vi "Do.vi"(8 "error in (no error)":errorcluster, 10 "Actor in":refnum<class "Actor.lvclass">, 11 "Stage Printing Loop Msg in":refnum<class "Stage Printing Loop Msg.lvclass">) -> (0 "error out":errorcluster, 2 "Actor out":refnum<class "Actor.lvclass">)   [LabVIEW 2018, in "Stage Printing Loop Msg.lvclass"]
doc: "This VI delivers the message to the actor by calling the appropriate method(s) on the actor."
uses:
  Stage Printing Loop Msg.lvclass
  <vilib>/ActorFramework/Actor/Actor.lvclass
  Stage/Stage.lvclass
  C:/Program Files/National Instruments/LabVIEW 2018/vi.lib/ActorFramework/Actor/Actor.lvclass
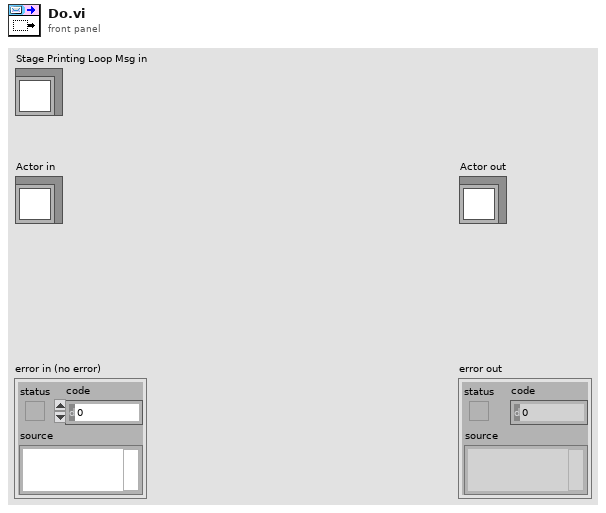
[diagram p1: front panel]
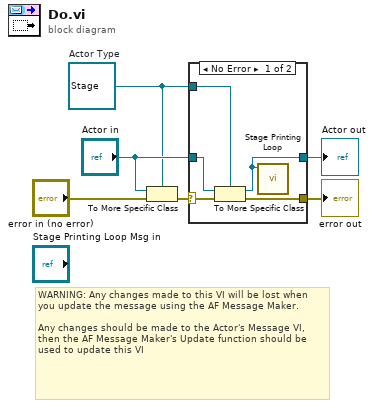
[diagram p0: block diagram]
diagram:
  w1 = refnum<class "Stage.lvclass"> refnum  # Actor Type
  # "WARNING: Any changes made to this VI will be lost when you update the message using the AF Message Maker.\n\nAny changes should be made to the Actor's Message VI, then the AF Message Maker's Update function should be used to update this VI"
  n1 = To More Specific Class(target class=w1, reference="Actor in", error in="error in (no error)") -> (error out=w5:errorcluster)  [unwired: 1 out]
  n2 = case shown="No Error" w5 {
    selector: w5 -> [w11 w13]
    tunnel: [w7 w13] -> w4
    tunnel: [w8 w12] -> w3
    tunnel: "Actor in" -> [w10 w12]
    tunnel: w1 -> [w9 _]
    frame No Error {
      n3 = To More Specific Class ("Actor Cast")(target class=w9, reference=w10, error in=w11) -> (specific class reference=w8:refnum<class "Stage.lvclass">, error out=w7:errorcluster)
      n4 = call "Stage Printing Loop.vi"("Stage Actor.lvlib:Stage.lvclass"=w8) -> ()  [unwired: 11 in]
    }
    frame Error {
    }
  }
  "error out" <- w4
  "Actor out" <- w3
